vi "Configure Marker State.vi"(7 "Marker On":bool, 8 "error in (no error)":errorcluster, 10 "Marker Number":u8=1, 11 "VNA-ENA in":refnum<class "VNA-ENA.lvclass">) -> (0 "error out":errorcluster, 3 "VNA-ENA out":refnum<class "VNA-ENA.lvclass">)   [LabVIEW 2020, in "VNA-ENA.lvclass"]
doc: "Configure the marker state.\nThe marker is on the active trace."
uses:
  VNA-ENA.lvclass
  C:/Sandbox/RF Bench/Source Code/WiSpry Test Framework/Instruments/Instrument.lvclass
  Instrument.lvclass/Instrument.ctl
  Instrument.lvclass
  <instrlib>/Agilent ENA Series/Agilent ENA Series.lvlib
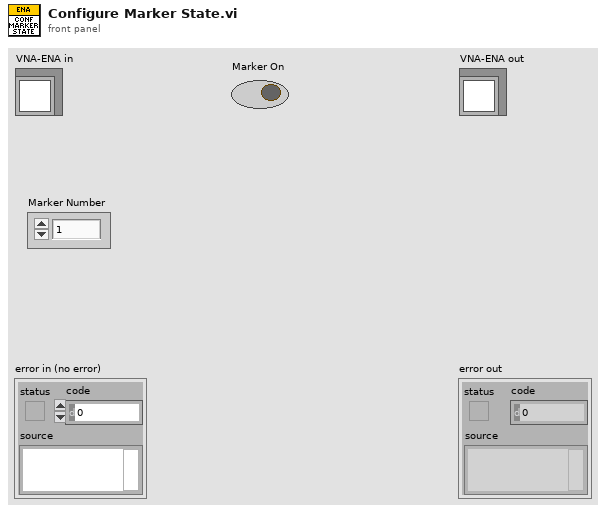
[diagram p1: front panel]
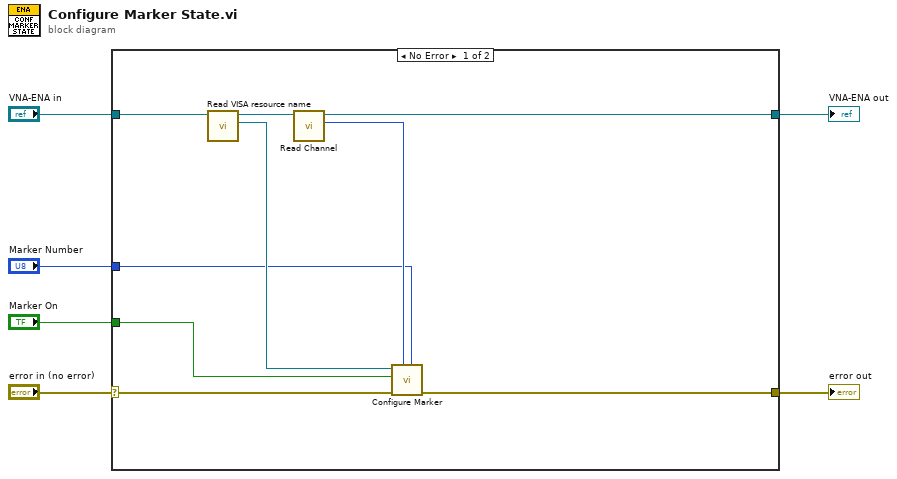
[diagram p0: block diagram]
diagram:
  n1 = case shown="No Error" "error in (no error)" {
    selector: "error in (no error)" -> [w8 w17]
    tunnel: [w7 w17] -> w5
    tunnel: [w14 w16] -> w4
    tunnel: "VNA-ENA in" -> [w15 w16]
    tunnel: "Marker Number" -> [w10 _]
    tunnel: "Marker On" -> [w9 _]
    frame No Error {
      n2 = call "Read VISA resource name.vi"("Instrument in"=w15) -> ("VISA resource name"=w12:refnum<visa-resource-name>, "Instrument out"=w13:refnum<class "VNA-ENA.lvclass">)  [unwired: 9 in]
      n3 = call-dynamic "Read Channel.vi"("Vector Network Analyzer in"=w13) -> ("Channel"=w11:i32, "Vector Network Analyzer out"=w14:refnum<class "VNA-ENA.lvclass">)  [unwired: 9 in]
      n4 = call <instrlib>:"Configure Marker.vi"("Marker (1)"=w10, "Channel (1)"=w11, "error in (no error)"=w8, "Marker State (F: Disabled)"=w9, "VISA resource name"=w12) -> ("error out"=w7:errorcluster)  [unwired: 5 in, 1 out]
    }
    frame Error {
    }
  }
  "error out" <- w5
  "VNA-ENA out" <- w4
